vi "Update_Status_Display.vi"(8 "error in (no error)":errorcluster, 10 "Status":string, 11 "DisplayConsole in":refnum<class "DisplayConsole.lvclass">) -> (0 "error out":errorcluster, 3 "DisplayConsole out":refnum<class "DisplayConsole.lvclass">)   [LabVIEW 2025, in "DisplayConsole.lvlib" / "DisplayConsole.lvclass"]
uses:
  DisplayConsole.lvclass
  DisplayConsole.lvclass/DisplayConsole.ctl
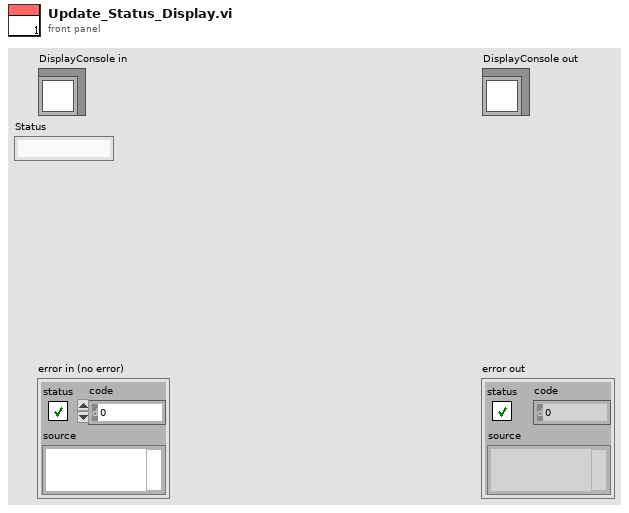
[diagram p1: front panel]
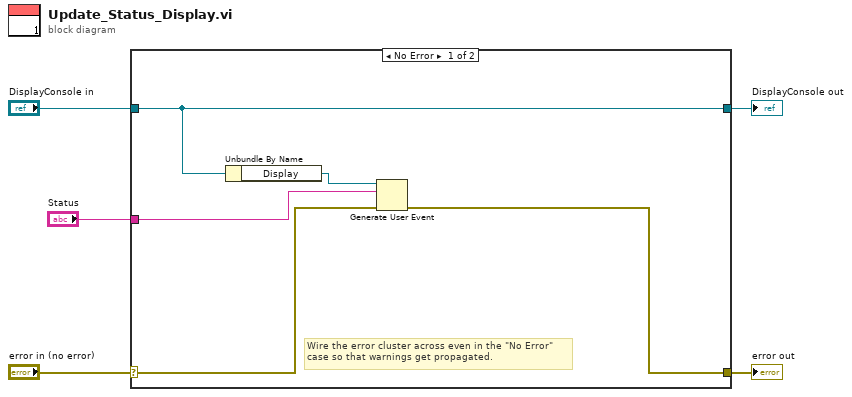
[diagram p0: block diagram]
diagram:
  n1 = case shown="No Error" "error in (no error)" {
    selector: "error in (no error)" -> [w8 w12]
    tunnel: [w7 w12] -> w4
    tunnel: [w10 w11] -> w2
    tunnel: "DisplayConsole in" -> [w10 w11]
    tunnel: "Status" -> [w6 _]
    frame No Error {
      # "Wire the error cluster across even in the \"No Error\"\ncase so that warnings get propagated."
      n2 = Unbundle By Name(w10) -> ("Display"=w9:refnum<user-event>)
      n3 = Generate User Event(user event=w9, event data cluster=w6, error in=w8) -> (error out=w7:errorcluster)  [unwired: 1 in, 1 out]
    }
    frame Error {
    }
  }
  "error out" <- w4
  "DisplayConsole out" <- w2
